vi "CleanUp.vi"(8 "Error In":errorcluster, 11 "object in":refnum<class "INI.lvclass">) -> (0 "Error Out":errorcluster, 3 "object out":refnum<class "INI.lvclass">)   [LabVIEW 2024]
uses:
  INI.lvclass/INI.ctl
  INI.lvclass
  C:/Apps/LVTimeTracker/LVTimeTracker/Projects/Parent/Projects.lvclass
  C:/Apps/LVTimeTracker/LVTimeTracker/Projects/INI_class/INI.lvclass
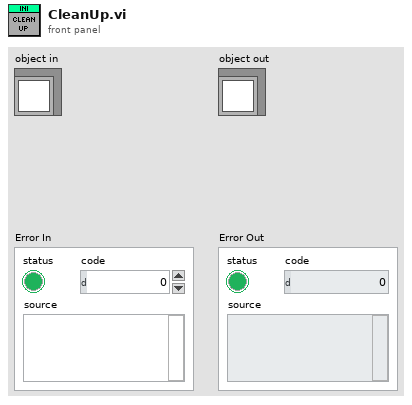
[diagram p1: front panel]
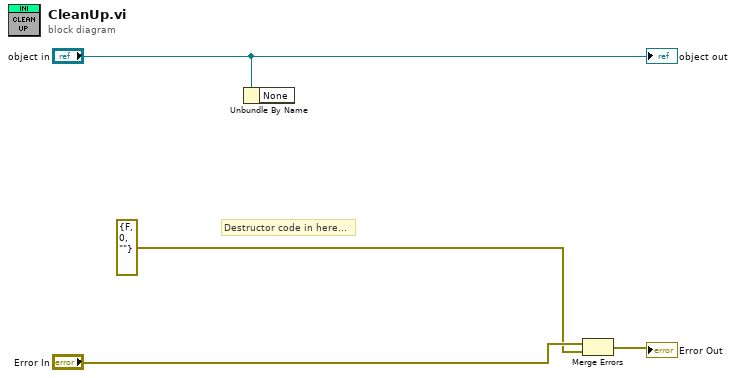
[diagram p0: block diagram]
diagram:
  # "Destructor code in here..."
  n1 = Unbundle By Name("object in") -> ()  [unwired: 1 out]
  n2 = Merge Errors("Error In", errorcluster {"status"=FALSE, "code"=0, "source"=""} ("error in (no error)")) -> (→"Error Out":errorcluster)
  "object out" <- "object in"
